vi "OE1311&OE1351_Configure Sensitivity and Filter.vi"(7 "OE1300_Configure \nSens and Filter":T1={"Time Constant(s) "=0.1, "Low Pass Filter Slope "=1, "Enable Sync Filter "=0, "Input Range"=2} {"Input Range" items=["5 V/uA", "2 V/uA", "1 V/uA", "500 mV/nA", "200 mV/nA", "100 mV/nA", "50 mV/nA", "20 mV/nA", "10 mV/nA", "5 mV/nA", "2 mV/nA", "1 mV/nA", "500 uV/pA", "200 uV/pA", "100 uV/pA", "50 uV/pA", "20 uV/pA", "10 uV/pA", "5 uV/pA", "2 uV/pA", "1 uV/pA", "500 nV/fA", "200 nV/fA", "100 nV/fA", "50 nV/fA", "20 nV/fA", "10 nV/fA", "5 nV/fA", "2 nV/fA", "1 nV/fA"]; "Enable Sync Filter" items=["OFF", "ON"]; "Low Pass Filter Slope" items=["6 dB/oct", "12 dB/oct", "18 db/oct", "24 dB/oct", "30 dB/oct", "36 dB/oct", "42 dB/oct", "48 dB/oct"]; "Time Constant(s)" min=1e-06 max=3000.0}, 8 "Error in (no error)":errorcluster caption="error out（no error）", 9 "Remote Mode":u16(ring)=1 items=["RS232"=1, "Ethernet"=3], 10 "Connection ID in":refnum<k5>, 11 "VISA resource name":refnum<visa-resource-name>) -> (0 "Error out":errorcluster caption="error out", 1 "Output String":string, 2 "Connection ID out":refnum<k5>, 3 "VISA resource  out":refnum<visa-resource-name>)   [LabVIEW 2011]
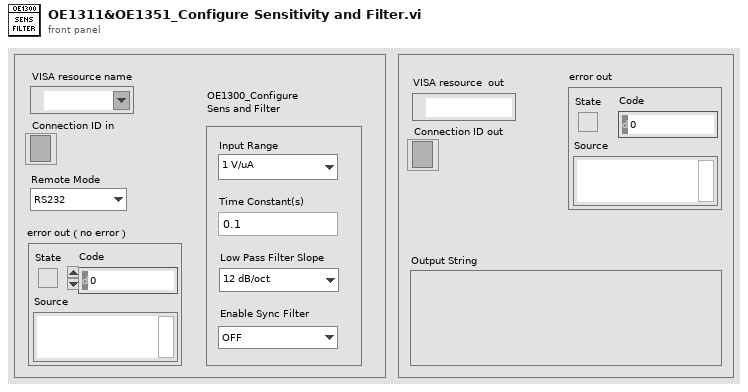
[diagram p1: front panel]
types:
  T1 = cluster{"Time Constant(s) ":dbl, "Low Pass Filter Slope ":u8, "Enable Sync Filter ":u16, "Input Range":u16}
  T2 = enum16{"ISRC", "IGND", "ICPL", "ILIN", "PHAS", "FMOD", "RSLP", "FREQ", "SWPT", "SLLM", "SULM", "SSLL", "SSLG", "STLM", "SWRM", "IRNG", "SENS", "RMOD", "OFLT", "OFSL", "SYNC", "DMOD", "HARM", "DARB", "SWVT", "SLVL", "SVLL", "SVUL", "SVSL", "SVSG", "SVTM", "SVRM", "RALL", "SNAP", "OUTP", "OAUX", "COUT", "CAUX", "COFP", "CEXP", "FPOP", "OEXP", "*IDN", "*RST", "OVLD", "INOV", "GNOV", "*PLL", "SSET", "RSET", "AGAN", "APHS", "ARSV", "ASCL", "EQCD", "EQCS", "SPED", "SRAT", "SLEN", "SSLE", "STRG", "SPRM", "STRD", "PAUS", "REST", "SPTS", "TRCA", "TEMP", "RSTU", "IHNZ", "DEQU", "SADD", "ARNG", "CSPE", "ISRCD", "IGNDD", "ICPLD", "ILIND", "PHASD", "FMODD", "RSLPD", "FREQD", "SWPTD", "SLLMD", "SULMD", "SSLLD", "SSLGD", "STLMD", "SWRMD", "SENSD", "RMODD", "OFLTD", "OFSLD", "SYNCD", "HARMD", "EQCDD", "EQCSD", "SNAPD", "OUTPD", "SWVTD", "SLVLD", "SVLLD", "SVULD", "SVSLD", "SVSGD", "SVTMD", "SVRMD", "SVDCD", "ARSVD", "AGAND", "APHSD", "ASCLD", "FPOPD", "CAUXD", "OEXPD", "SPEDD", "SRATD", "SLEND", "SSLED", "STRGD", "SPRMD", "STRDD", "PAUSD", "RESTD", "SPTSD", "TRCAD", "*IDND", "*RSTD", "INOVD", "GNOVD", "*PLLD", "SSETD", "RSETD"}
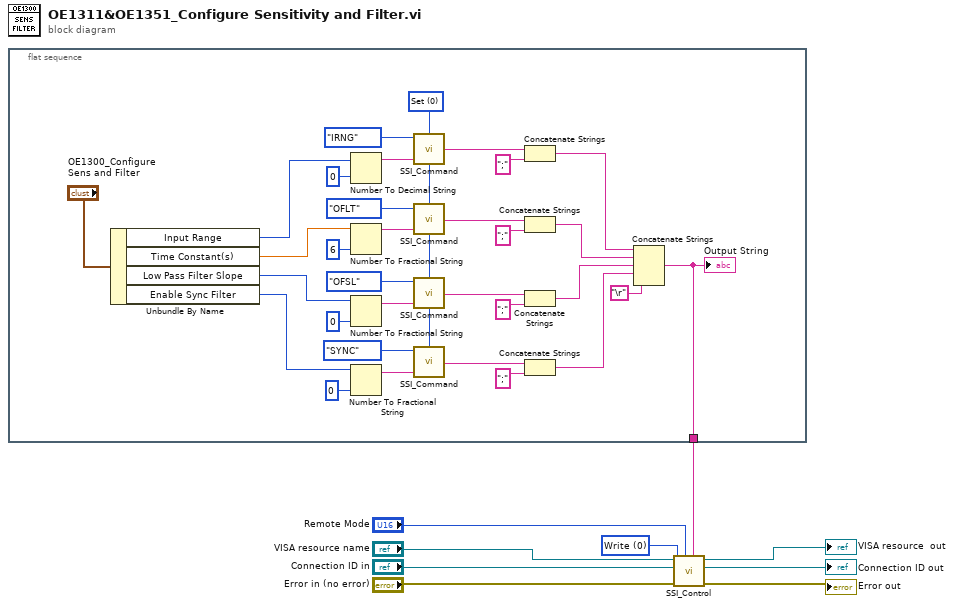
[diagram p0: block diagram]
diagram:
  w7 = u16 0 items=["Write", "Read"] ("Control")
  n1 = flat-sequence {
    tunnel: [w11] -> w1
    frame #0 {
      w18 = u16 0 items=["Set", "Query"] ("Opera")
      n2 = Unbundle By Name("OE1300_Configure \nSens and Filter") -> ("Input Range"=w27:u16, "Time Constant(s)"=w26:dbl, "Low Pass Filter Slope"=w25:u8, "Enable Sync Filter"=w17:u16)
      n3 = Number To Decimal String(number=w27, width (-)=i16 0 ("宽度(-)")) -> (decimal integer string=w41:string)
      n4 = Number To Fractional String(number=w26, precision (6)=i16 6 ("宽度(-)")) -> (F-format string=w39:string)  [unwired: 2 in]
      n5 = Number To Fractional String(number=w25, precision (6)=i16 0 ("精度(6)")) -> (F-format string=w37:string)  [unwired: 2 in]
      n6 = Number To Fractional String(number=w17, precision (6)=i16 0 ("精度(6)")) -> (F-format string=w22:string)  [unwired: 2 in]
      n7 = call "SSI_Command.vi"("Opera"=w18, "Paramter"=w41, "Command Type"=T2."IRNG") -> ("Output string"=w34:string)  [unwired: 1 in]
      n8 = call "SSI_Command.vi"("Opera"=w18, "Paramter"=w39, "Command Type"=T2."OFLT") -> ("Output string"=w30:string)  [unwired: 1 in]
      n9 = call "SSI_Command.vi"("Opera"=w18, "Paramter"=w37, "Command Type"=T2."OFSL") -> ("Output string"=w32:string)  [unwired: 1 in]
      n10 = call "SSI_Command.vi"("Opera"=w18, "Paramter"=w22, "Command Type"=T2."SYNC") -> ("Output string"=w19:string)  [unwired: 1 in]
      n11 = Concatenate Strings(w34, ";" ("替换字符串(\"\")")) -> (w29:string)
      n12 = Concatenate Strings(w30, ";" ("替换字符串(\"\")")) -> (w24:string)
      n13 = Concatenate Strings(w32, ";" ("替换字符串(\"\")")) -> (w23:string)
      n14 = Concatenate Strings(w19, ";" ("替换字符串(\"\")")) -> (w12:string)
      n15 = Concatenate Strings(w29, w24, w23, w12, "\r") -> (w11:string)
      "Output String" <- w11
    }
  }
  n16 = call "SSI_Control.vi"("Write Buffer"=w1, "Remote Mode"="Remote Mode", "Error in (no error)"="Error in (no error)", "Control"=w7, "Connection ID in"="Connection ID in", "VISA resource name"="VISA resource name") -> ("Error out"=→"Error out":errorcluster, "Connection ID out"=→"Connection ID out":refnum<k5>, "VISA resource  out"=→"VISA resource  out":refnum<visa-resource-name>)  [unwired: 2 in, 1 out]
